vi "Spawner.vi"(8 "error in (no error)":errorcluster, 10 "Map":i32[](array[numeric]), 11 "Spawner In":refnum<class "Cross.lvclass">) -> (0 "error out":errorcluster, 1 "Direction":T1, 2 "Action":T2, 3 "Spawner Out":refnum<class "Cross.lvclass">, 4 "Replicated Class":refnum<class "Cross.lvclass">)   [LabVIEW 2015, in "Cross.lvclass"]
uses:
  Cross.lvclass
  Type Defs/Action Enum.ctl
  Type Defs/Direction Enum.ctl
  Cross.lvclass/Cross.ctl
  Type Defs/SB Type Defs.lvlib
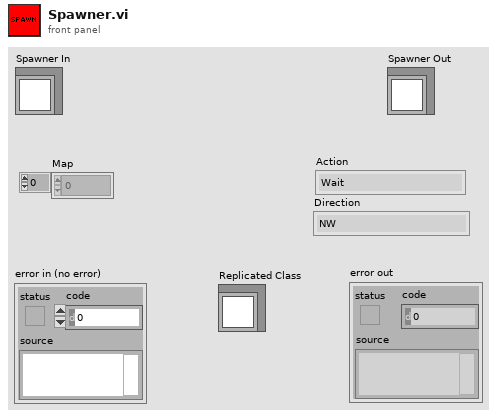
[diagram p1: front panel]
types:
  T1 = typedef "SB Type Defs.lvlib/Direction Enum.ctl" = enum16{"NW", "N", "NE", "E", "SE", "S", "SW", "W"}
  T2 = typedef "SB Type Defs.lvlib/Action Enum.ctl" = enum16{"Wait", "Move", "Attack", "Replicate"}
  T3 = enum16{"Raw", "Spawner", "Builder", "Gunner", "Fighter"}
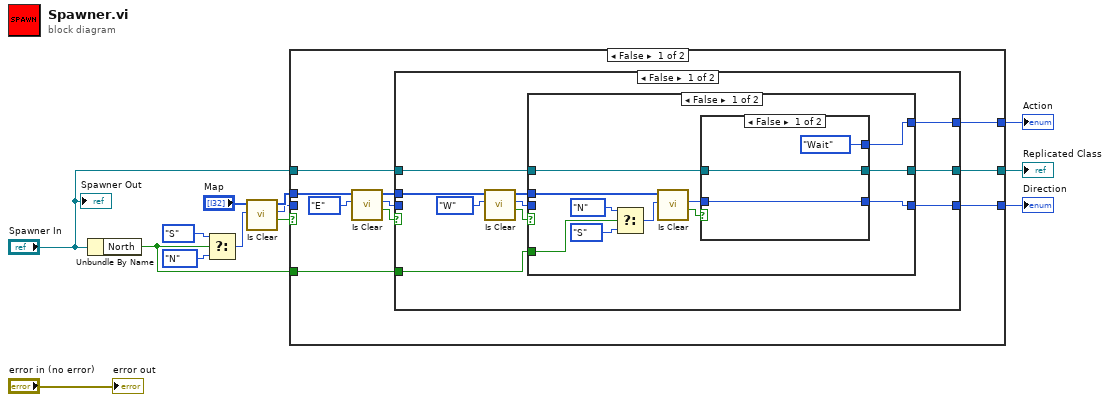
[diagram p0: block diagram]
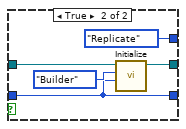
[diagram p2: hidden frame]
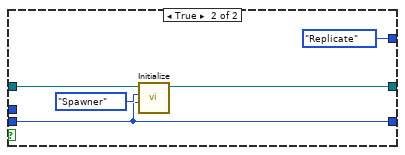
[diagram p3: hidden frame]
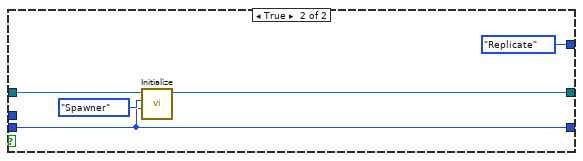
[diagram p4: hidden frame]
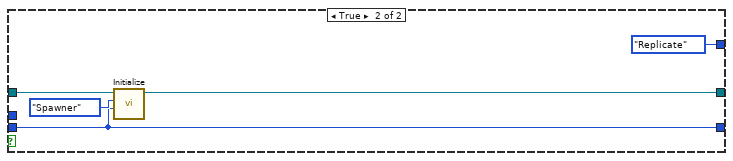
[diagram p5: hidden frame]
diagram:
  n1 = Unbundle By Name("Spawner In") -> ("North"=w1:bool)
  n2 = Select(t=Direction_Enum."S" ("Direction"), s=w1, f=Direction_Enum."N" ("Direction")) -> (s? t:f=w6:T1)
  n3 = call "Is Clear.vi"("Direction"=w6, "Maze"="Map") -> ("Can Move?"=w4:bool, "Direction Out"=w3:T1, "Maze"=w5:i32[])  [unwired: 6 in, 1 out]
  n4 = case shown="False" w4 {
    tunnel: [w17 Action_Enum."Replicate" ("Action")] -> w10
    tunnel: "Spawner In" -> [w14 w64]
    tunnel: [w16 w65] -> w8
    tunnel: w5 -> [w20 _]
    tunnel: w3 -> [_ w63]
    tunnel: [w15 w63] -> w2
    tunnel: w1 -> [w18 _]
    frame False {
      n5 = call "Is Clear.vi"("Direction"=Direction_Enum."E", "Maze"=w20) -> ("Can Move?"=w21:bool, "Direction Out"=w22:T1, "Maze"=w19:i32[])  [unwired: 6 in, 1 out]
      n6 = case shown="False" w21 {
        tunnel: w22 -> [_ w58]
        tunnel: w19 -> [w32 _]
        tunnel: w18 -> [w28 _]
        tunnel: [w27 Action_Enum."Replicate" ("Action")] -> w17
        tunnel: [w26 w60] -> w16
        tunnel: [w25 w58] -> w15
        tunnel: w14 -> [w24 w61]
        frame False {
          n7 = call "Is Clear.vi"("Direction"=Direction_Enum."W", "Maze"=w32) -> ("Can Move?"=w30:bool, "Direction Out"=w29:T1, "Maze"=w31:i32[])  [unwired: 6 in, 1 out]
          n8 = case shown="False" w30 {
            tunnel: w31 -> [w36 _]
            tunnel: w29 -> [_ w56]
            tunnel: w28 -> [w38 _]
            tunnel: [w43 Action_Enum."Replicate" ("Action")] -> w27
            tunnel: [w42 w53] -> w26
            tunnel: [w41 w56] -> w25
            tunnel: w24 -> [w40 w54]
            frame False {
              n9 = Select(t=Direction_Enum."N" ("Direction"), s=w38, f=Direction_Enum."S" ("Direction")) -> (s? t:f=w37:T1)
              n10 = call "Is Clear.vi"("Direction"=w37, "Maze"=w36) -> ("Can Move?"=w34:bool, "Direction Out"=w35:T1)  [unwired: 6 in, 2 out]
              n11 = case shown="False" w34 {
                tunnel: w40 -> [w46 w49]
                tunnel: w35 -> [w45 w48]
                tunnel: [Action_Enum."Wait" ("Action") Action_Enum."Replicate" ("Action")] -> w43
                tunnel: [w46 w50] -> w42
                tunnel: [w45 w48] -> w41
                frame False {
                }
                frame True {
                  n12 = call "Initialize.vi"("Direction"=w48, "Job"=T3."Builder", "Runner in"=w49) -> ("Runner out"=w50:refnum<class "Cross.lvclass">)  [unwired: 8 in]
                }
              }
            }
            frame True {
              n13 = call "Initialize.vi"("Direction"=w56, "Job"=T3."Spawner", "Runner in"=w54) -> ("Runner out"=w53:refnum<class "Cross.lvclass">)  [unwired: 8 in]
            }
          }
        }
        frame True {
          n14 = call "Initialize.vi"("Direction"=w58, "Job"=T3."Spawner", "Runner in"=w61) -> ("Runner out"=w60:refnum<class "Cross.lvclass">)  [unwired: 8 in]
        }
      }
    }
    frame True {
      n15 = call "Initialize.vi"("Direction"=w63, "Job"=T3."Spawner", "Runner in"=w64) -> ("Runner out"=w65:refnum<class "Cross.lvclass">)  [unwired: 8 in]
    }
  }
  "Action" <- w10
  "Direction" <- w2
  "Replicated Class" <- w8
  "error out" <- "error in (no error)"
  "Spawner Out" <- "Spawner In"
